vi "FeedbackDecode_CopyRemoteFiles.vi"(3 "DataFolder":string, 4 "CompName":string, 5 "Mode":enum16{"Decode", "Encode"}(ring)) -> (0 "OrigName":string, 2 "MLName":string)   [LabVIEW 2020]
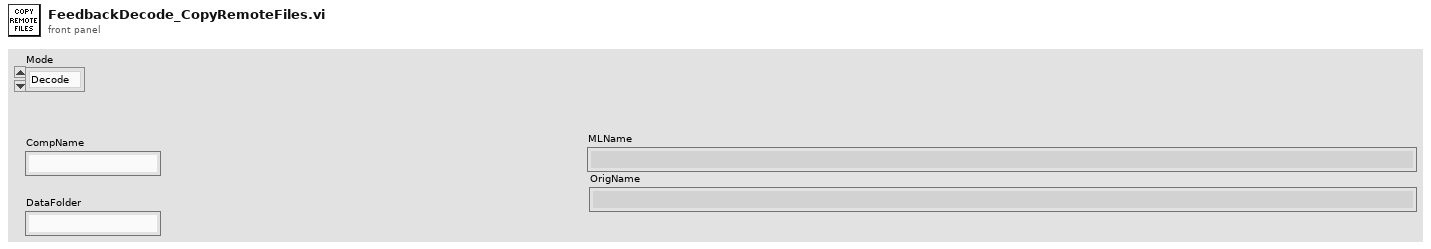
[diagram p1: front panel]
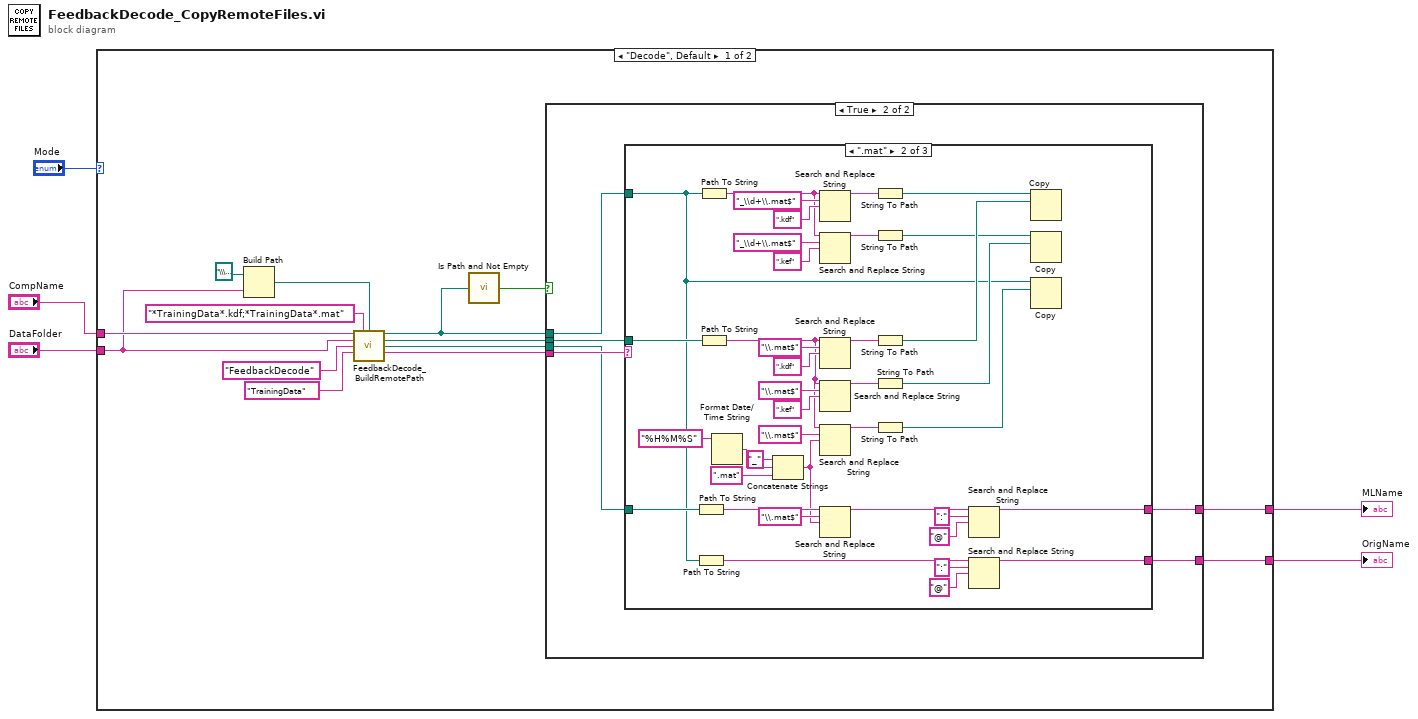
[diagram p0: block diagram]
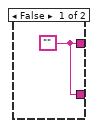
[diagram p2: hidden frame]
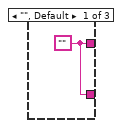
[diagram p3: hidden frame]
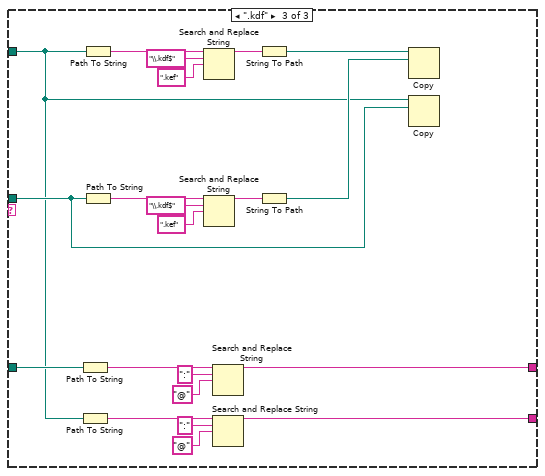
[diagram p4: hidden frame]
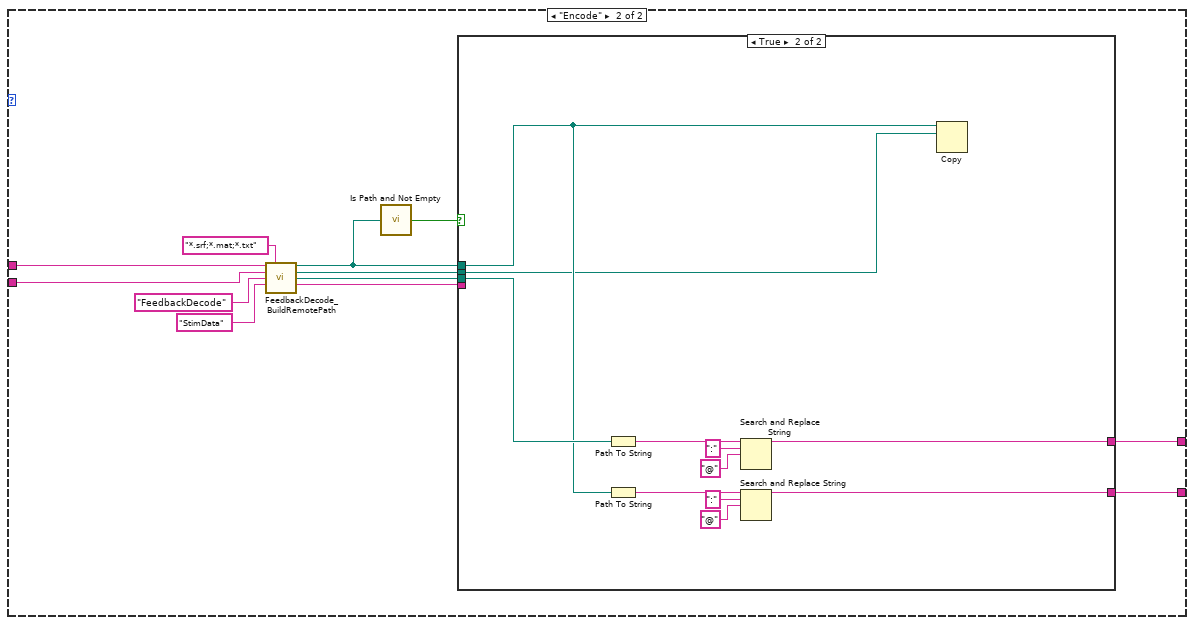
[diagram p5: hidden frame]
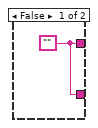
[diagram p6: hidden frame]
diagram:
  n1 = case shown="\"Decode\", Default" "Mode" {
    tunnel: [w12 w92] -> w5
    tunnel: [w11 w91] -> w4
    tunnel: "CompName" -> [w9 w89]
    tunnel: "DataFolder" -> [w8 w88]
    frame "Decode", Default {
      n2 = Build Path(base path=path "\\\\pnimatlab\\PNIMatlab_R1/FeedbackDecode", name or relative path=w8) -> (appended path=w7:path)
      n3 = call "FeedbackDecode_BuildRemotePath.vi"("CompName"=w9, "FilePattern"="*TrainingData*.kdf;*TrainingData*.mat" ("pattern (all files)"), "StartPath"=w7, "DataFolder"=w8, "TaskName"="FeedbackDecode", "HeaderName"="TrainingData" ("TaskName")) -> ("OriginalName"=w13:path, "RemoteNetName"=w15:path, "RemoteLocalName"=w14:path, "FileExt"=w16:string)  [unwired: 5 in, 1 out]
      n4 = call <vilib>:"Is Path and Not Empty.vi"("path"=w13) -> ("Is Path and Not Empty?"=w10:bool)  [unwired: 4 in]
      n5 = case shown="True" w10 {
        tunnel: w16 -> [_ w26]
        tunnel: w15 -> [_ w25]
        tunnel: w14 -> [_ w24]
        tunnel: w13 -> [_ w23]
        tunnel: [w20 w22] -> w12
        tunnel: [w20 w21] -> w11
        frame False {
          w20 = ""
        }
        frame True {
          n6 = case shown="\".mat\"" w26 {
            tunnel: w23 -> [_ w34 w69]
            tunnel: w25 -> [_ w48 w73]
            tunnel: w24 -> [_ w43 w77]
            tunnel: [w27 w29 w68] -> w22
            tunnel: [w27 w28 w67] -> w21
            frame "", Default {
              w27 = ""
            }
            frame ".mat" {
              n7 = Path To String(path=w43) -> (string=w32:string)
              n8 = Path To String(path=w34) -> (string=w37:string)
              n9 = Path To String(path=w34) -> (string=w62:string)
              n10 = Path To String(path=w48) -> (string=w47:string)
              n11 = Format Date/Time String(time format string (%c)="%H%M%S") -> (date/time string=w50:string)  [unwired: 2 in]
              n12 = Concatenate Strings("_" ("string"), w50, ".mat" ("string")) -> (w31:string)
              n13 = Search and Replace String(input string=w62, search string="_\\d+\\.mat$" ("regular expression"), replace string=".kdf" ("replace string (\"\")")) -> (result string=w61:string)  [unwired: 5 in, 3 out]
              n14 = Search and Replace String(input string=w62, search string="_\\d+\\.mat$" ("regular expression"), replace string=".kef" ("replace string (\"\")")) -> (result string=w60:string)  [unwired: 5 in, 3 out]
              n15 = Search and Replace String(input string=w47, search string="\\.mat$" ("regular expression"), replace string=".kdf" ("replace string (\"\")")) -> (result string=w59:string)  [unwired: 5 in, 3 out]
              n16 = Search and Replace String(input string=w47, search string="\\.mat$" ("regular expression"), replace string=".kef" ("replace string (\"\")")) -> (result string=w54:string)  [unwired: 5 in, 3 out]
              n17 = Search and Replace String(input string=w47, search string="\\.mat$" ("regular expression"), replace string=w31) -> (result string=w51:string)  [unwired: 5 in, 3 out]
              n18 = Search and Replace String(input string=w32, search string="\\.mat$" ("regular expression"), replace string=w31) -> (result string=w30:string)  [unwired: 5 in, 3 out]
              n19 = String To Path(string=w61) -> (path=w42:path)
              n20 = String To Path(string=w60) -> (path=w40:path)
              n21 = String To Path(string=w59) -> (path=w41:path)
              n22 = String To Path(string=w54) -> (path=w39:path)
              n23 = String To Path(string=w51) -> (path=w38:path)
              n24 = Search and Replace String(input string=w30, search string=":", replace string="@" ("replace string (\"\")")) -> (result string=w29:string)  [unwired: 5 in, 3 out]
              n25 = Search and Replace String(input string=w37, search string=":", replace string="@" ("replace string (\"\")")) -> (result string=w28:string)  [unwired: 5 in, 3 out]
              n26 = Copy(10:w41, 11:w42) -> ()  [unwired: 3 in, 3 out]
              n27 = Copy(10:w39, 11:w40) -> ()  [unwired: 3 in, 3 out]
              n28 = Copy(10:w38, 11:w34) -> ()  [unwired: 3 in, 3 out]
            }
            frame ".kdf" {
              n29 = Path To String(path=w77) -> (string=w76:string)
              n30 = Path To String(path=w69) -> (string=w72:string)
              n31 = Path To String(path=w69) -> (string=w85:string)
              n32 = Path To String(path=w73) -> (string=w80:string)
              n33 = Search and Replace String(input string=w85, search string="\\.kdf$" ("regular expression"), replace string=".kef" ("replace string (\"\")")) -> (result string=w84:string)  [unwired: 5 in, 3 out]
              n34 = Search and Replace String(input string=w80, search string="\\.kdf$" ("regular expression"), replace string=".kef" ("replace string (\"\")")) -> (result string=w83:string)  [unwired: 5 in, 3 out]
              n35 = Search and Replace String(input string=w76, search string=":", replace string="@" ("replace string (\"\")")) -> (result string=w68:string)  [unwired: 5 in, 3 out]
              n36 = Search and Replace String(input string=w72, search string=":", replace string="@" ("replace string (\"\")")) -> (result string=w67:string)  [unwired: 5 in, 3 out]
              n37 = String To Path(string=w84) -> (path=w75:path)
              n38 = String To Path(string=w83) -> (path=w74:path)
              n39 = Copy(10:w74, 11:w75) -> ()  [unwired: 3 in, 3 out]
              n40 = Copy(10:w73, 11:w69) -> ()  [unwired: 3 in, 3 out]
            }
          }
        }
      }
    }
    frame "Encode" {
      n41 = call "FeedbackDecode_BuildRemotePath.vi"("CompName"=w89, "FilePattern"="*.srf;*.mat;*.txt" ("pattern (all files)"), "DataFolder"=w88, "TaskName"="FeedbackDecode", "HeaderName"="StimData" ("TaskName")) -> ("OriginalName"=w93:path, "RemoteNetName"=w95:path, "RemoteLocalName"=w94:path, "FileExt"=w96:string)  [unwired: 6 in, 1 out]
      n42 = call <vilib>:"Is Path and Not Empty.vi"("path"=w93) -> ("Is Path and Not Empty?"=w90:bool)  [unwired: 4 in]
      n43 = case shown="True" w90 {
        tunnel: w96 -> [_ _]
        tunnel: w95 -> [_ w101]
        tunnel: w94 -> [_ w111]
        tunnel: w93 -> [_ w102]
        tunnel: [w100 w110] -> w92
        tunnel: [w100 w109] -> w91
        frame False {
          w100 = ""
        }
        frame True {
          n44 = Path To String(path=w111) -> (string=w106:string)
          n45 = Path To String(path=w102) -> (string=w105:string)
          n46 = Search and Replace String(input string=w106, search string=":", replace string="@" ("replace string (\"\")")) -> (result string=w110:string)  [unwired: 5 in, 3 out]
          n47 = Search and Replace String(input string=w105, search string=":", replace string="@" ("replace string (\"\")")) -> (result string=w109:string)  [unwired: 5 in, 3 out]
          n48 = Copy(10:w101, 11:w102) -> ()  [unwired: 3 in, 3 out]
        }
      }
    }
  }
  "MLName" <- w5
  "OrigName" <- w4
